vi "Get IDs.vi"(8 "error in (no error)":errorcluster, 11 "IHandleSubscribed in":refnum<class "IHandleSubscribed.lvclass">) -> (0 "error out":errorcluster, 1 "Subscription ID":u64, 2 "Subscription Request ID":u64, 3 "IHandleSubscribed out":refnum<class "IHandleSubscribed.lvclass">)   [LabVIEW 2020, in "wamplv.lvlib" / "IHandleSubscribed.lvclass"]
uses:
  IHandleSubscribed.lvclass
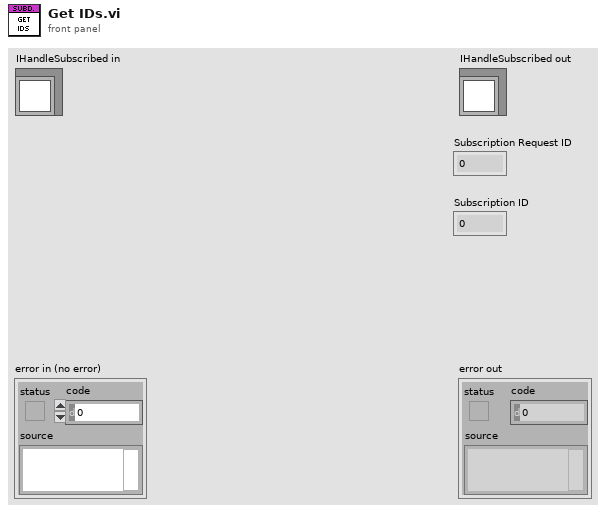
[diagram p1: front panel]
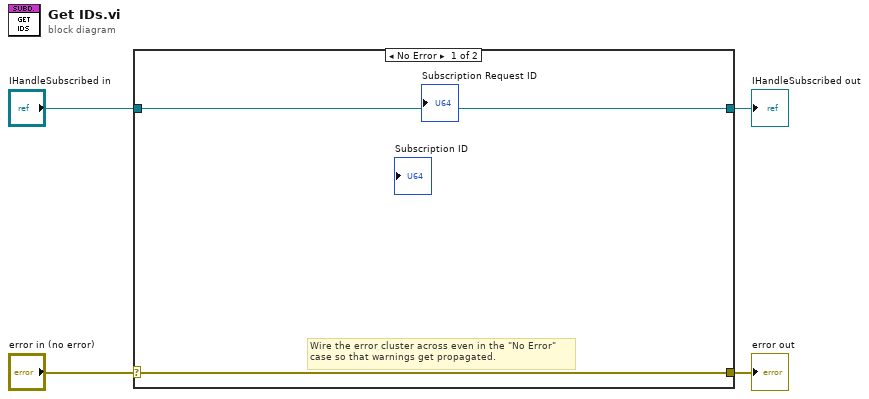
[diagram p0: block diagram]
diagram:
  n1 = case shown="No Error" "error in (no error)" {
    selector: "error in (no error)" -> [w5 w8]
    tunnel: [w5 w8] -> w3
    tunnel: [w6 w7] -> w1
    tunnel: "IHandleSubscribed in" -> [w6 w7]
    frame No Error {
      # "Wire the error cluster across even in the \"No Error\"\ncase so that warnings get propagated."
    }
    frame Error {
    }
  }
  "error out" <- w3
  "IHandleSubscribed out" <- w1
